vi "Waveform to Cluster.vi"(1 "Waveform":waveform(dbl)(graph)) -> (0 "Clustered  Wave":cluster{"Y":dbl[], dbl[]})   [LabVIEW 2018]
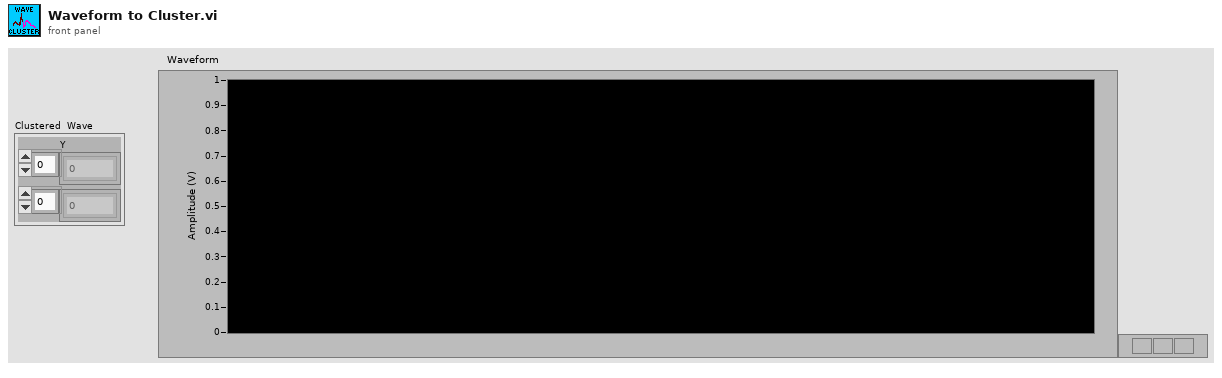
[diagram p1: front panel]
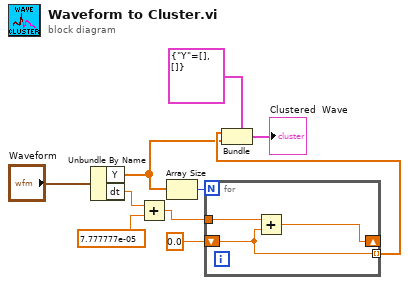
[diagram p0: block diagram]
diagram:
  n1 = Unbundle By Name("Waveform") -> ("Y"=w4:dbl[], "dt"=w3:dbl)
  n2 = Add(x=w3, y=7.777777e-05) -> (x+y=w1:dbl)
  n3 = Array Size(array=w4) -> (size(s)=w9:i32)
  n4 = for {
    N: w9 -> [_]
    tunnel: w1 -> [w13]
    shift-right: [w12] -> _
    shift-left: 0.0 -> [w11]
    tunnel: [w11] -> w5 mode=indexing
    n5 = Add(x=w13, y=w11) -> (x+y=w12:dbl)
  }
  n6 = Bundle(cluster=cluster{"Y":dbl[], dbl[]} {"Y"=[], []}, "Y"=w5, w4) -> (→"Clustered  Wave":cluster{"Y":dbl[], dbl[]})
